vi "BCD To Number.vi"(0 "BCD":u16) -> (6 "Number":u16)   [LabVIEW 2024]
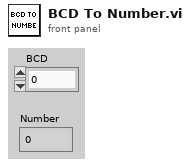
[diagram p1: front panel]
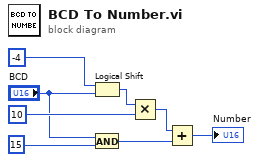
[diagram p0: block diagram]
diagram:
  n1 = Logical Shift(y=i16 -4, x="BCD") -> (x << y=w7:u16)
  n2 = And(x="BCD", y=u16 15) -> (x .and. y?=w3:u16)
  n3 = Multiply(x=w7, y=u16 10) -> (x*y=w2:u16)
  n4 = Add(x=w2, y=w3) -> (x+y=→"Number":u16)
